vi "Apply Synch.vi"(8 "error in":errorcluster, 11 "4300 in":refnum<class "4300.lvclass">) -> (0 "error out":errorcluster, 3 "4300 out":refnum<class "4300.lvclass">)   [LabVIEW 2019, in "4300.lvlib" / "4300.lvclass"]
uses:
  Library/4300.lvclass
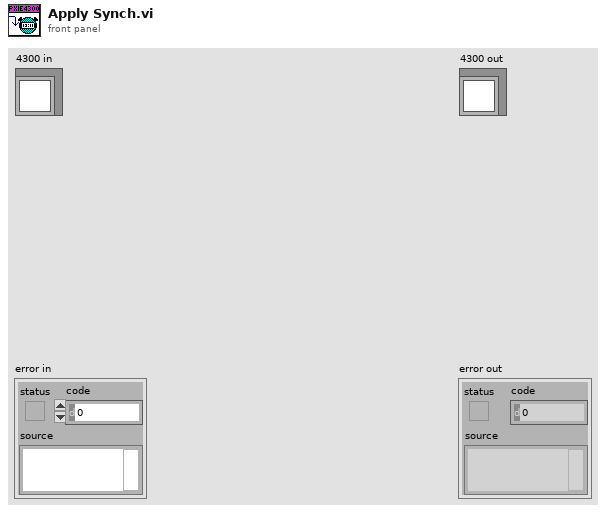
[diagram p1: front panel]
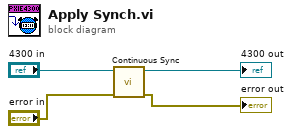
[diagram p0: block diagram]
diagram:
  n1 = call "Continuous Sync.vi"("error in"="error in", "4300 in"="4300 in") -> ("error out"=→"error out":errorcluster, "4300 out"=→"4300 out":refnum<class "4300.lvclass">)  [unwired: 8 in]
